vi "Utility_RW String to Local Drive.vi"(5 "File Name":string="4296 Data", 7 "System":string="4296 Data", 8 "Error":errorcluster, 9 "Read(f)Write(t)":bool, 10 "Data Name":string="VisonSettings", 11 "String Data":string) -> (0 "Error Out":errorcluster, 2 "Found? Out":bool, 3 "String Data Out":string)   [LabVIEW 2017]
doc: "This example shows how to use the Configuration File VIs to save key-value pairs to, and read key-value pairs from, an ini file on the robot.\n\nThis example expects a USB cable connected from your development PC to the Type B USB Jack (next to the power input) on the roboRIO."
uses:
  <vilib>/Utility/config.llb/Read Key (String).vi
  <vilib>/Utility/config.llb/Write Key (String).vi
  <vilib>/Utility/config.llb/NI_LVConfig.lvlib
  <vilib>/Utility/sysdir.llb/System Directory Type.ctl
panel:
  out "File Path Out":path
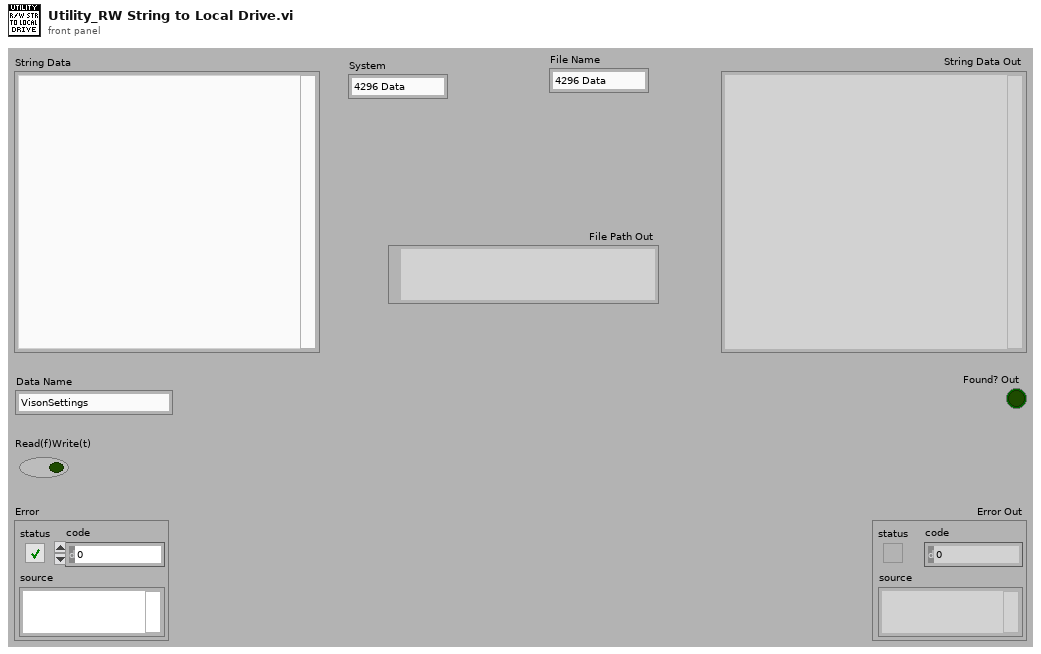
[diagram p1: front panel]
types:
  T1 = typedef "System Directory Type.ctl" = i32
  T2 = typedef "NI_LVConfig.lvlib/Config Data RefNum.ctl" = refnum<k1>
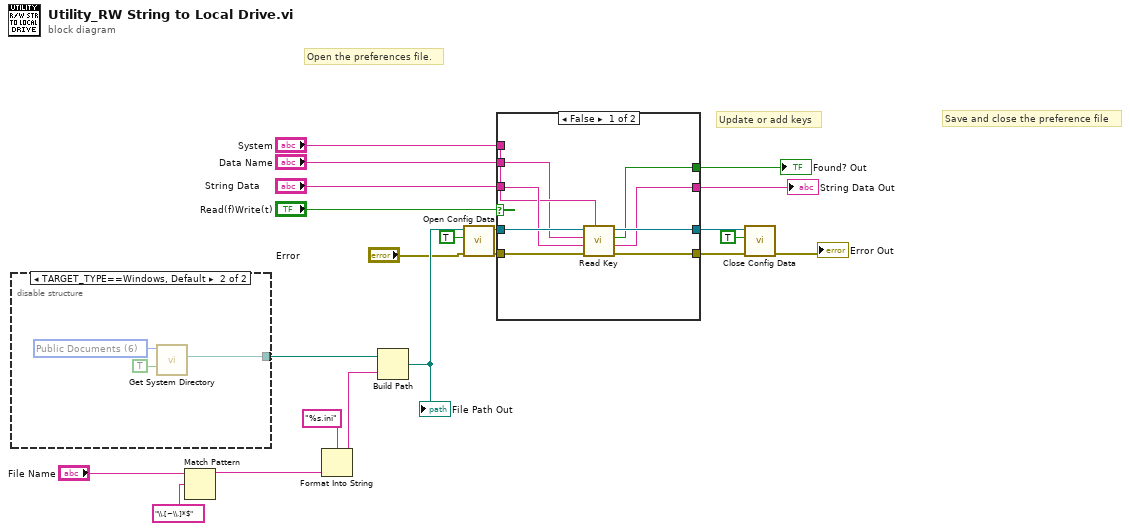
[diagram p0: block diagram]
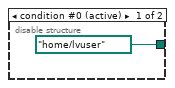
[diagram p2: hidden frame]
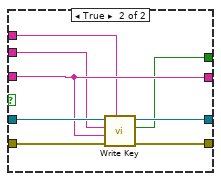
[diagram p3: hidden frame]
diagram:
  # "Save and close the preference file"
  # "Update or add keys"
  # "Open the preferences file."
  n1 = disable-structure shown="TARGET_TYPE==Windows, Default" {
    disable-tunnel: [path "/home/lvuser" ("configuration file path") w23] -> w13
    frame condition #0 (active) {
    }
    frame condition #1 {
      w25 = T1 6 items=["User Home"=0, "User Desktop"=1, "User Documents"=2, "User Application Data"=3, "User Preferences"=4, "User Temporary"=5, "Public Documents"=6, "Public Application Data"=7, "Public Preferences"=8, "Public Cache"=13, "System Core Libraries"=9, "System Installed Libraries"=10, "Application Files"=11, "Boot Volume Root"=12] ("system directory type")
      n2 = call <vilib>:"Get System Directory.vi"("create directory if not found? (F)"=TRUE, "system directory type"=w25) -> ("system directory"=w23:path)  [unwired: 9 in]
    }
  }
  n3 = Match Pattern(string="File Name", regular expression="\\.[~\\.]*$") -> (before substring=w7:string)  [unwired: 4 out]
  n4 = Format Into String(format string="%s.ini", w7) -> (resulting string=w11:string)  [unwired: 2 in, 1 out]
  n5 = Build Path(base path=w13, name or relative path=w11) -> (appended path=w14:path)
  "File Path Out" <- w14
  n6 = call <vilib>:"Open Config Data.vi"("error in (no error)"="Error", "create file if necessary (T)"=TRUE, "configuration file path"=w14) -> ("error out"=w5:errorcluster, "refnum"=w21:T2)  [unwired: 6 in, 1 out]
  n7 = case shown="False" "Read(f)Write(t)" {
    tunnel: w21 -> [w34 w42]
    tunnel: "Data Name" -> [w26 w35]
    tunnel: [w33 w41] -> w19
    tunnel: [w32 w40] -> w18
    tunnel: [w31 w39] -> w17
    tunnel: "String Data" -> [w28 w40]
    tunnel: w5 -> [w30 w38]
    tunnel: [w29 w37] -> w4
    tunnel: "System" -> [w27 w36]
    frame False {
      n8 = call-poly <vilib>:"Read Key.vi"("section"=w27, "error in (no error)"=w30, "default value"=w28, "key"=w26, "refnum"=w34) -> ("error out"=w29:errorcluster, "value"=w32:string, "found?"=w31:bool, "refnum out"=w33:T2)  [unwired: 3 in]
    }
    frame True {
      n9 = call-poly <vilib>:"Write Key.vi"("section"=w36, "error in (no error)"=w38, "value"=w40, "key"=w35, "refnum"=w42) -> ("error out"=w37:errorcluster, "found?"=w39:bool, "refnum out"=w41:T2)  [unwired: 4 in]
    }
  }
  "String Data Out" <- w18
  "Found? Out" <- w17
  n10 = call <vilib>:"Close Config Data.vi"("error in (no error)"=w4, "write file if changed (T)"=TRUE, "refnum"=w19) -> ("error out"=→"Error Out":errorcluster)  [unwired: 7 in, 1 out]
